vi "Configure Self Calibrate Lock.vi"(8 "error in (no error)":errorcluster, 10 "Lock Balance Self Calibration":bool caption="Lock Balance Self Calibration (F: Unlock)", 11 "VISA resource name":refnum<visa-resource-name>) -> (0 "error out":errorcluster, 3 "VISA resource name out":refnum<visa-resource-name>)   [LabVIEW 2017, in "RadWag balances and scales.lvlib"]
doc: "Confiigures the lock balances internal calibration.\nInternal calibration are proceeded after internally seted time and/or after internally setted operating temperature change.\nThis VI stops balances from internal calibrating, although when balance is verified internal calibration can not be locked."
uses:
  <instrlib>/Prev/RadWag Continuous Read Folder/RadWag balances and scales.lvlib
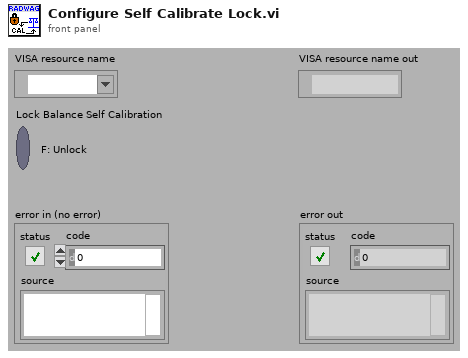
[diagram p1: front panel]
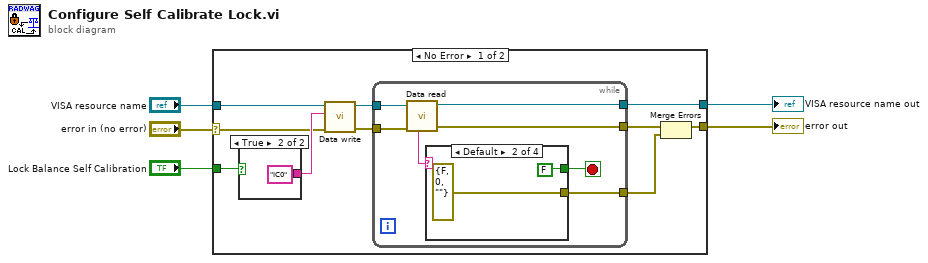
[diagram p0: block diagram]
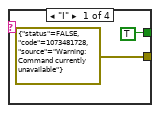
[diagram p2: hidden frame]
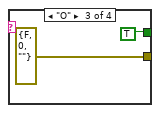
[diagram p3: hidden frame]
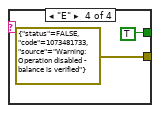
[diagram p4: hidden frame]
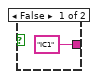
[diagram p5: hidden frame]
diagram:
  n1 = case shown="No Error" "error in (no error)" {
    selector: "error in (no error)" -> [w9 w33]
    tunnel: [w15 w34] -> w5
    tunnel: [w7 w33] -> w4
    tunnel: "VISA resource name" -> [w14 w34]
    tunnel: "Lock Balance Self Calibration" -> [w13 _]
    frame No Error {
      n2 = case shown="True" w13 {
        tunnel: ["IC1" ("ID") "IC0" ("ID")] -> w10
        frame False {
        }
        frame True {
        }
      }
      n3 = call <instrlib>:"Data write.vi"("error in (no error)"=w9, "ID"=w10, "VISA resource name"=w14) -> ("error out"=w11:errorcluster, "VISA resource name out"=w12:refnum<visa-resource-name>)  [unwired: 7 in]
      n4 = while {
        tunnel: w12 -> [w22]
        tunnel: [w21] -> w15
        tunnel: w11 -> [w20]
        tunnel: [w19] -> w8
        tunnel: [w16] -> w6
        stop <- w17 stop-if-true
        n5 = call <instrlib>:"Data read.vi"("error in (no error)"=w20, "VISA resource name"=w22) -> ("error out"=w19:errorcluster, "VISA resource name out"=w21:refnum<visa-resource-name>, "Status"=w18:string)  [unwired: 3 in, 4 out]
        n6 = case shown="Default" w18 {
          tunnel: [errorcluster {"status"=FALSE, "code"=1073481728, "source"="Warning: Command currently unavailable"} ("t") errorcluster {"status"=FALSE, "code"=0, "source"=""} ("error constant") errorcluster {"status"=FALSE, "code"=0, "source"=""} ("error constant") errorcluster {"status"=FALSE, "code"=1073481733, "source"="Warning: Operation disabled - balance is verified"} ("t")] -> w16
          tunnel: [TRUE FALSE TRUE TRUE] -> w17
          frame "I" {
          }
          frame Default {
          }
          frame "O" {
          }
          frame "E" {
          }
        }
      }
      n7 = Merge Errors(w8, w6) -> (w7:errorcluster)
    }
    frame Error {
    }
  }
  "error out" <- w4
  "VISA resource name out" <- w5
